vi "Actor Core.vi"(8 "error in":errorcluster, 11 "Optimization in":refnum<class "Optimization.lvclass">) -> (0 "error out":errorcluster, 3 "Actor out":refnum<class "Actor.lvclass">)   [LabVIEW 2016, in "Optimization Framework.lvlib" / "Optimization.lvclass"]
doc: "(<B>Filename</B>: Actor Framework.lvlib:Actor.lvclass:Actor Core.vi)\n\nReceives messages to the actor, reacts to them, and initiates any error handling that may shut the actor down.\n\nDescendant classes may override this VI to append parallel tasks for the actor to complete while it handles messages. Overrides use the Call Parent Method node."
uses:
  Optimization.lvclass
  C:/Program Files (x86)/National Instruments/LabVIEW 2016/vi.lib/ActorFramework/Actor/Actor.lvclass
  <vilib>/ActorFramework/Actor/Actor.lvclass
  Controls/Microgrid State Selector.ctl
  Utilities/Delivery Notifier Handler.llb/Delivery Notifier Handler Command.ctl
  Optimization.lvclass/Optimization.ctl
  <vilib>/ActorFramework/Message Enqueuer/Message Enqueuer.lvclass/Message Enqueuer.ctl
  Commissioning Actor/Commissioning/Commissioning.lvclass
  Activation Actor/Activation/Activation.lvclass
  Blackstart Actor/Blackstart/Blackstart.lvclass
  On-Grid Actor/On-Grid/On-Grid.lvclass
  Off-Grid Actor/Off-Grid/Off-Grid.lvclass
  Island Actor/Island/Island.lvclass
  Resynchronization Actor/Resynchronization/Resynchronization.lvclass
  Shutdown Actor/Shutdown/Shutdown.lvclass
  <vilib>/ActorFramework/Stop Msg/Send Normal Stop.vi
  <vilib>/Utility/error.llb/Clear Errors.vi
  <vilib>/ActorFramework/Message Enqueuer/Enqueue.vi
  <vilib>/ActorFramework/Stop Msg/Stop Msg.lvclass
  C:/Program Files (x86)/National Instruments/LabVIEW 2016/vi.lib/ActorFramework/Message/Message.lvclass
  <vilib>/ActorFramework/Message Priority Queue/Priority Enqueue.vi
  Global Variables/Global Variables.vi
  <vilib>/ActorFramework/Message Enqueuer/Message Enqueuer.lvclass
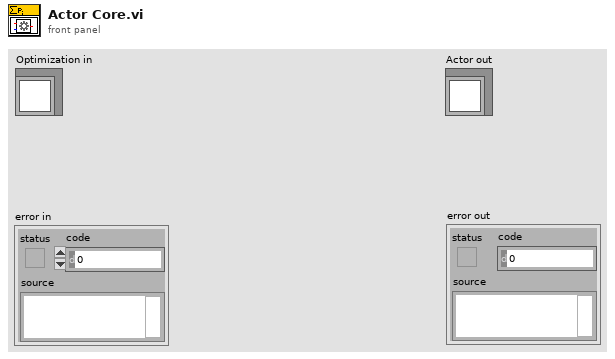
[diagram p1: front panel]
types:
  T1 = typedef "Optimization Framework.lvlib/Optimization.lvclass/Delivery Notifier Handler Command.ctl" = enum16{"Initiate", "Store", "Close All"}
  T2 = typedef "Optimization Framework.lvlib/Optimization.lvclass/Microgrid State Selector.ctl" = enum16{"Invalid", "Commissioning", "Activation", "Blackstart", "OnGrid", "OffGrid", "Islanding", "Resynchronization", "Shutdown"}
  T3 = typedef "Optimization Framework.lvlib/Optimization.lvclass/Optimization User Events.ctl" = cluster{"Microgrid State":refnum<user-event>, "stop":refnum<user-event>}
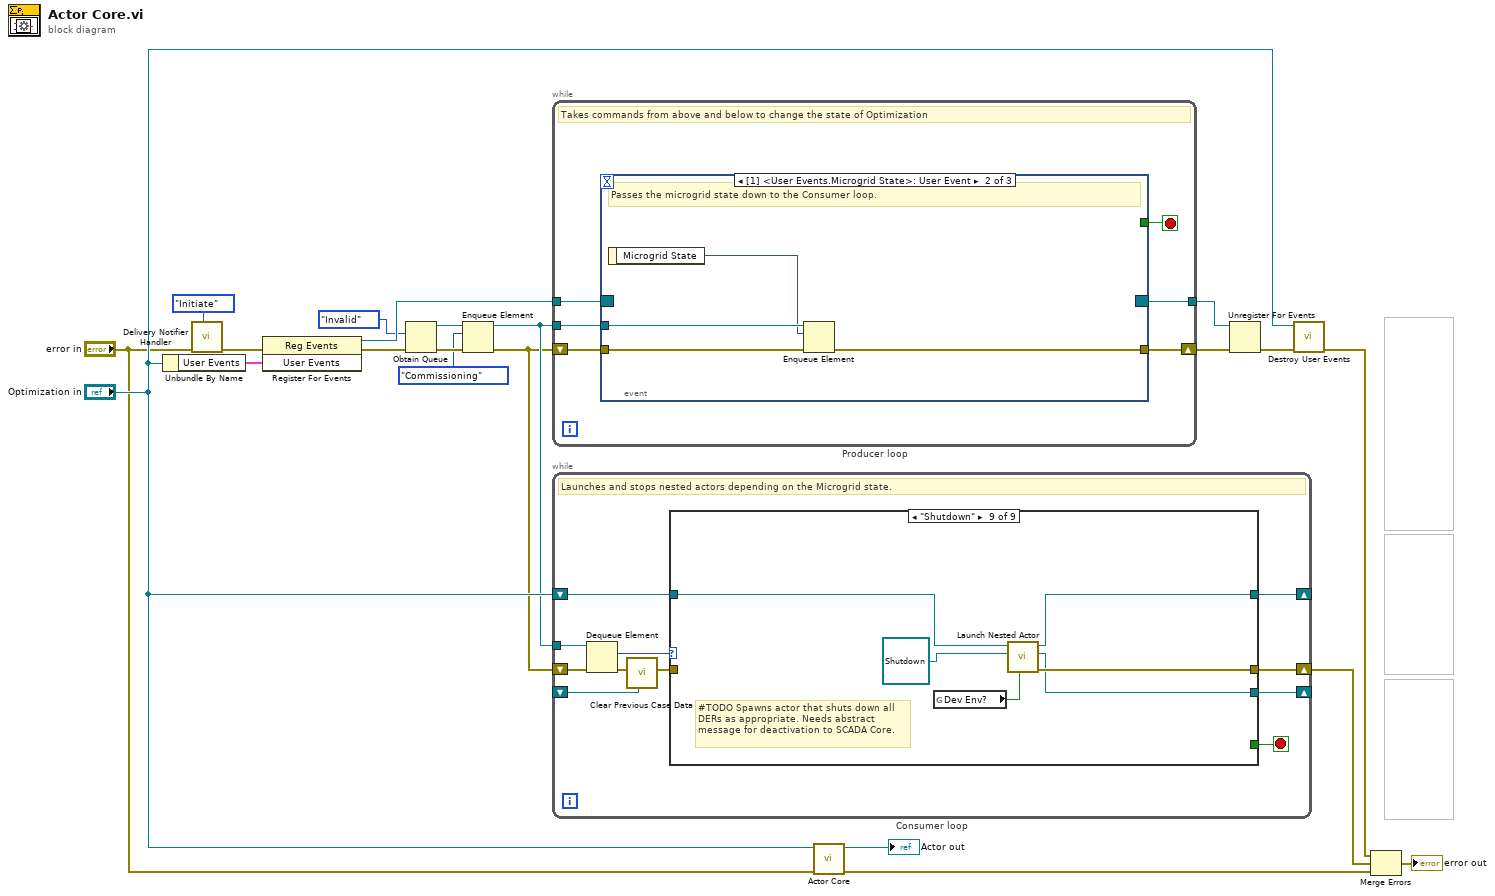
[diagram p0: block diagram]
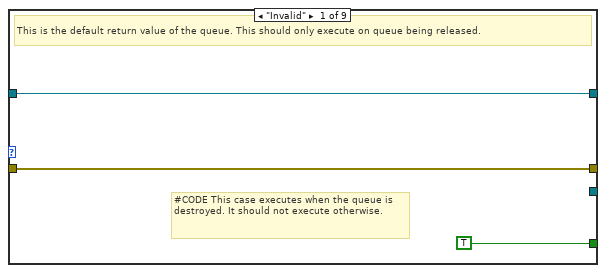
[diagram p2: hidden frame]
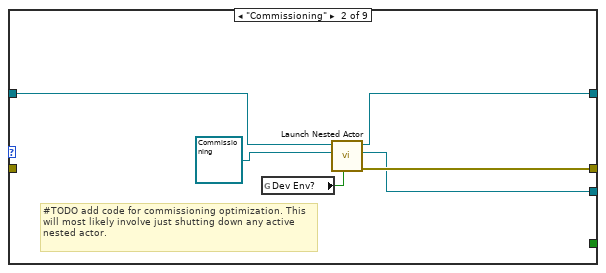
[diagram p3: hidden frame]
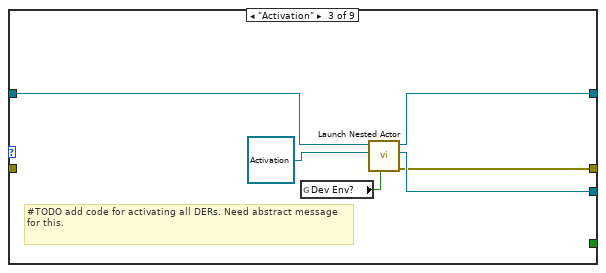
[diagram p4: hidden frame]
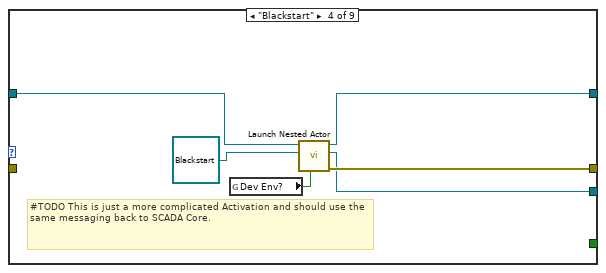
[diagram p5: hidden frame]
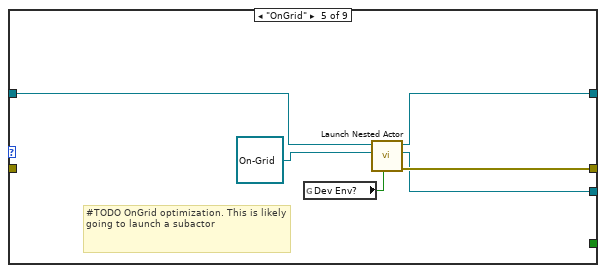
[diagram p6: hidden frame]
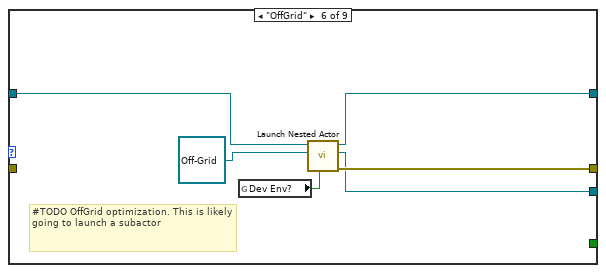
[diagram p7: hidden frame]
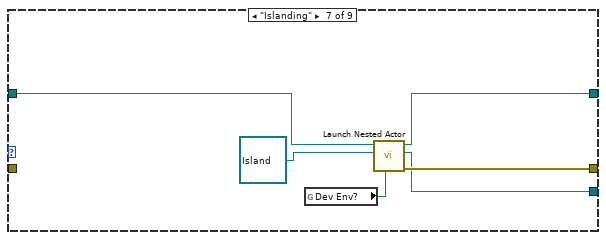
[diagram p8: hidden frame]
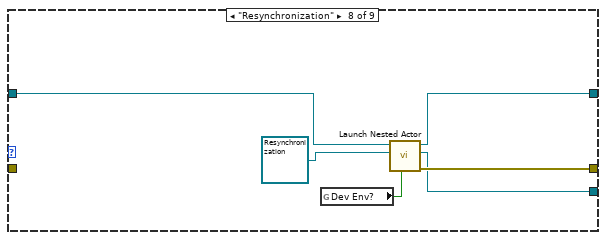
[diagram p9: hidden frame]
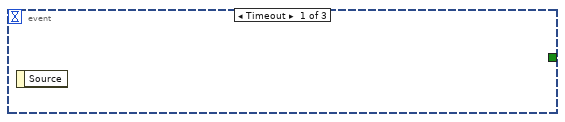
[diagram p10: hidden frame]
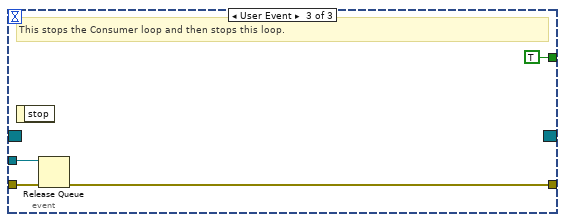
[diagram p11: hidden frame]
diagram:
  n1 = Unbundle By Name("Optimization in") -> ("User Events"=w19:T3)
  n2 = call "Delivery Notifier Handler.vi"("Command (Store)"=Delivery_Notifier_Handler_Command."Initiate", "error in"="error in") -> ("error out"=w2:errorcluster)  [unwired: 9 in]
  n3 = register-events(error in=w2, w19) -> (reference out=w18:refnum<event-registration>, error out=w15:errorcluster)  [unwired: 1 in]
  n4 = Obtain Queue(element data type=Microgrid_State_Selector."Invalid" ("Microgrid State"), error in (no error)=w15) -> (queue out=w16:refnum<queue>, error out=w6:errorcluster)  [unwired: 3 in, 1 out]
  n5 = Enqueue Element(queue=w16, element=Microgrid_State_Selector."Commissioning", error in (no error)=w6) -> (queue out=w7:refnum<queue>, error out=w5:errorcluster)  [unwired: 1 in, 1 out]
  n6 = while "Producer loop" {
    tunnel: w7 -> [w27]
    tunnel: w18 -> [w26]
    shift-right: [w24] -> w14
    shift-left: w5 -> [w25]
    tunnel: [w23] -> w12
    stop <- w22 stop-if-true
    # "Takes commands from above and below to change the state of Optimization"
    n7 = event shown="[1] <User Events.Microgrid State>: User Event" {
      selector: w26 -> [_ _ _]
      dyn-events: [_ _ _] -> w23
      timeout: _ -> [_ _ _]
      tunnel: w27 -> [_ w31 w33]
      tunnel: w25 -> [_ w29 w34]
      tunnel: [_ w28 w32] -> w24
      tunnel: [_ _ TRUE] -> w22
      event Timeout {
        n8 = event-data() -> ()  [unwired: 1 in, 1 out]
      }
      event User Event {
        # "Passes the microgrid state down to the Consumer loop."
        n9 = event-data() -> ("Microgrid State"=w30:T2)  [unwired: 1 in]
        n10 = Enqueue Element(queue=w31, element=w30, error in (no error)=w29) -> (error out=w28:errorcluster)  [unwired: 1 in, 2 out]
      }
      event User Event {
        # "This stops the Consumer loop and then stops this loop."
        n11 = event-data() -> ()  [unwired: 1 in, 1 out]
        n12 = Release Queue(queue=w33, error in (no error)=w34) -> (error out=w32:errorcluster)  [unwired: 1 in, 2 out]
      }
    }
  }
  n13 = while "Consumer loop" {
    tunnel: w7 -> [w46]
    shift-right: [w44] -> w9
    shift-left: w5 -> [w45]
    shift-right: [w40] -> _
    shift-left: "Optimization in" -> [w41]
    shift-right: [w39] -> _
    shift-left: _ -> [w36]
    stop <- w42 stop-if-true
    # "Launches and stops nested actors depending on the Microgrid state."
    n14 = Dequeue Element(queue=w46, error in (no error)=w45) -> (element=w43:T2, error out=w38:errorcluster)  [unwired: 1 in, 2 out]
    n15 = call "Clear Previous Case Data.vi"("Nested Actor's Enqueuer"=w36, "error in"=w38) -> ("error out"=w37:errorcluster)  [unwired: 9 in]
    n16 = case shown="\"Shutdown\"" w43 {
      tunnel: w37 -> [w49 _ _ _ _ _ _ _ _]
      tunnel: [w49 w55 w59 w67 w73 w77 w85 w91 w97] -> w44
      tunnel: [TRUE _ _ _ _ _ _ _ _] -> w42
      tunnel: w41 -> [w47 w52 w58 w66 w69 w78 w81 w87 w94]
      tunnel: [w47 w54 w61 w65 w72 w79 w84 w89 w95] -> w40
      tunnel: [_ w53 w60 w64 w71 w76 w83 w90 w96] -> w39
      frame "Invalid" {
        # "#CODE This case executes when the queue is destroyed. It should not execute otherwise."
        # "This is the default return value of the queue. This should only execute on queue being released."
      }
      frame "Commissioning" {
        # "#TODO add code for commissioning optimization. This will most likely involve just shutting down any active nested actor."
        n17 = global read "Global Variables.vi" "Dev Env?"() -> (w50:bool)
        n18 = call <vilib>:"Launch Nested Actor.vi"("Open Actor Core front panel? (F)"=w50, "Nested Actor"=refnum<class "Commissioning.lvclass"> refnum ("Commissioning Actor.lvlib:Commissioning.lvclass"), "Caller Actor in"=w52) -> ("error out"=w55:errorcluster, "Nested Actor's Enqueuer"=w53:refnum<class "Message Enqueuer.lvclass">, "Caller Actor out"=w54:refnum<class "Optimization.lvclass">)  [unwired: 6 in]
      }
      frame "Activation" {
        # "#TODO add code for activating all DERs. Need abstract message for this."
        n19 = global read "Global Variables.vi" "Dev Env?"() -> (w56:bool)
        n20 = call <vilib>:"Launch Nested Actor.vi"("Open Actor Core front panel? (F)"=w56, "Nested Actor"=refnum<class "Activation.lvclass"> refnum ("Activation in"), "Caller Actor in"=w58) -> ("error out"=w59:errorcluster, "Nested Actor's Enqueuer"=w60:refnum<class "Message Enqueuer.lvclass">, "Caller Actor out"=w61:refnum<class "Optimization.lvclass">)  [unwired: 6 in]
      }
      frame "Blackstart" {
        # "#TODO This is just a more complicated Activation and should use the same messaging back to SCADA Core."
        n21 = global read "Global Variables.vi" "Dev Env?"() -> (w62:bool)
        n22 = call <vilib>:"Launch Nested Actor.vi"("Open Actor Core front panel? (F)"=w62, "Nested Actor"=refnum<class "Blackstart.lvclass"> refnum ("Blackstart Actor.lvlib:Blackstart.lvclass"), "Caller Actor in"=w66) -> ("error out"=w67:errorcluster, "Nested Actor's Enqueuer"=w64:refnum<class "Message Enqueuer.lvclass">, "Caller Actor out"=w65:refnum<class "Optimization.lvclass">)  [unwired: 6 in]
      }
      frame "OnGrid" {
        # "#TODO OnGrid optimization. This is likely going to launch a subactor"
        n23 = global read "Global Variables.vi" "Dev Env?"() -> (w68:bool)
        n24 = call <vilib>:"Launch Nested Actor.vi"("Open Actor Core front panel? (F)"=w68, "Nested Actor"=refnum<class "On-Grid.lvclass"> refnum ("On-Grid Actor.lvlib:On-Grid.lvclass"), "Caller Actor in"=w69) -> ("error out"=w73:errorcluster, "Nested Actor's Enqueuer"=w71:refnum<class "Message Enqueuer.lvclass">, "Caller Actor out"=w72:refnum<class "Optimization.lvclass">)  [unwired: 6 in]
      }
      frame "OffGrid" {
        # "#TODO OffGrid optimization. This is likely going to launch a subactor"
        n25 = global read "Global Variables.vi" "Dev Env?"() -> (w74:bool)
        n26 = call <vilib>:"Launch Nested Actor.vi"("Open Actor Core front panel? (F)"=w74, "Nested Actor"=refnum<class "Off-Grid.lvclass"> refnum ("Off-Grid in"), "Caller Actor in"=w78) -> ("error out"=w77:errorcluster, "Nested Actor's Enqueuer"=w76:refnum<class "Message Enqueuer.lvclass">, "Caller Actor out"=w79:refnum<class "Optimization.lvclass">)  [unwired: 6 in]
      }
      frame "Islanding" {
        n27 = global read "Global Variables.vi" "Dev Env?"() -> (w80:bool)
        n28 = call <vilib>:"Launch Nested Actor.vi"("Open Actor Core front panel? (F)"=w80, "Nested Actor"=refnum<class "Island.lvclass"> refnum ("Island in"), "Caller Actor in"=w81) -> ("error out"=w85:errorcluster, "Nested Actor's Enqueuer"=w83:refnum<class "Message Enqueuer.lvclass">, "Caller Actor out"=w84:refnum<class "Optimization.lvclass">)  [unwired: 6 in]
      }
      frame "Resynchronization" {
        n29 = global read "Global Variables.vi" "Dev Env?"() -> (w86:bool)
        n30 = call <vilib>:"Launch Nested Actor.vi"("Open Actor Core front panel? (F)"=w86, "Nested Actor"=refnum<class "Resynchronization.lvclass"> refnum ("Resynchronization in"), "Caller Actor in"=w87) -> ("error out"=w91:errorcluster, "Nested Actor's Enqueuer"=w90:refnum<class "Message Enqueuer.lvclass">, "Caller Actor out"=w89:refnum<class "Optimization.lvclass">)  [unwired: 6 in]
      }
      frame "Shutdown" {
        # "#TODO Spawns actor that shuts down all DERs as appropriate. Needs abstract message for deactivation to SCADA Core."
        n31 = global read "Global Variables.vi" "Dev Env?"() -> (w92:bool)
        n32 = call <vilib>:"Launch Nested Actor.vi"("Open Actor Core front panel? (F)"=w92, "Nested Actor"=refnum<class "Shutdown.lvclass"> refnum ("Shutdown in"), "Caller Actor in"=w94) -> ("error out"=w97:errorcluster, "Nested Actor's Enqueuer"=w96:refnum<class "Message Enqueuer.lvclass">, "Caller Actor out"=w95:refnum<class "Optimization.lvclass">)  [unwired: 6 in]
      }
    }
  }
  n33 = call-parent "Actor Core.vi"("error in"="error in", "Actor in"="Optimization in") -> ("error out"=w21:errorcluster, "Actor out"=→"Actor out":refnum<class "Actor.lvclass">)  [unwired: 8 in]
  n34 = Unregister For Events(event registration refnum=w12, error in=w14) -> (error out=w13:errorcluster)
  n35 = call "Destroy User Events.vi"("error in"=w13, "Optimization in"="Optimization in") -> ("error out"=w10:errorcluster)  [unwired: 8 in, 1 out]
  n36 = Merge Errors(w10, w9, w21) -> (→"error out":errorcluster)
